vi "DHE_get_auto_shutter_clear.vi"(8 "error in (no error)":errorcluster, 11 "fd":i32) -> (0 "error out":errorcluster, 1 "autoshutter":bool, 2 "autoclear":bool, 3 "fd out":i32)   [LabVIEW 2016]
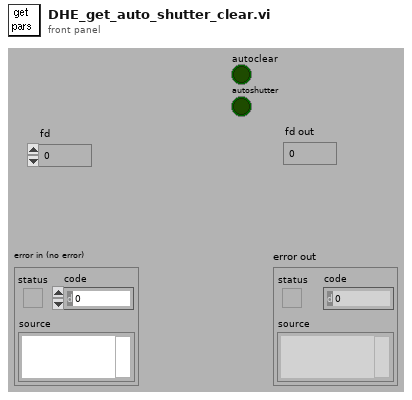
[diagram p1: front panel]
types:
  T1 = typedef "CMN_ContStatus.ctl" = cluster{"Response":string, "power":bool, "shutter":bool, "artifdata":bool, "idlemode":bool, "reset":bool, "gain":i32, "speed":i32, "resetPCI":bool, "autoshutter":bool, "TempSetPoint":i32, "multipleextensions":bool, "displayImage":bool, "coadding":bool, "images being coadded":i32, "Operation Mode":enum16{"normal", "coadd", "fawler"}, "frames to write":cluster{"subs":bool, "reset":bool, "exposed":bool}, "fawler samples":i32, "write auto":bool, "datatype":string, "frames to display":cluster{"subs":bool, "reset":bool, "exposed":bool}, "sur":i32, "autoclear":bool}
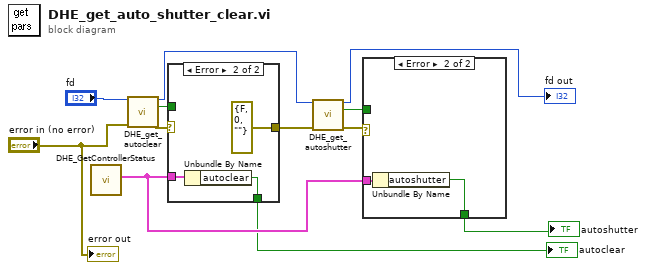
[diagram p0: block diagram]
diagram:
  n1 = call "DHE_GetControllerStatus.vi"() -> ("ControllerStatus"=w4:T1)  [unwired: 11 out]
  n2 = call "DHE_get_autoclear.vi"("fd in"="fd", "error in (no error)"="error in (no error)") -> ("fd out"=w8:i32, "autoclear"=w10:bool, "error out"=w11:errorcluster)  [unwired: 11 out]
  n3 = case shown="Error" w11 {
    selector: w11 -> [w13 _]
    tunnel: w10 -> [w14 _]
    tunnel: w4 -> [_ w17]
    tunnel: [w14 w16] -> w2
    tunnel: [w13 errorcluster {"status"=FALSE, "code"=0, "source"=""} ("error IO")] -> w9
    frame No Error {
    }
    frame Error {
      n4 = Unbundle By Name(w17) -> ("autoclear"=w16:bool)
    }
  }
  "autoclear" <- w2
  n5 = call "DHE_get_autoshutter.vi"("fd in"=w8, "error in (no error)"=w9) -> ("fd out"=→"fd out":i32, "autoshutter"=w6:bool, "error out"=w7:errorcluster)  [unwired: 11 out]
  n6 = case shown="Error" w7 {
    tunnel: w6 -> [w18 _]
    tunnel: [w18 w19] -> w1
    tunnel: w4 -> [_ w20]
    frame No Error {
    }
    frame Error {
      n7 = Unbundle By Name(w20) -> ("autoshutter"=w19:bool)
    }
  }
  "autoshutter" <- w1
  "error out" <- "error in (no error)"
